vi "SetCategoryHierarchy.vi"(8 "error in (no error)":errorcluster, 9 "Category hierarchy[]":string[](array[string]), 11 "CLabVIEWItem in":refnum<class "CLabVIEWItem.lvclass">) -> (0 "error out":errorcluster, 3 "CLabVIEWItem out":refnum<class "CLabVIEWItem.lvclass">)   [LabVIEW 2020, in "LabVIEWItem.lvlib" / "CLabVIEWItem.lvclass"]
uses:
  CLabVIEWItem.lvclass
  CLabVIEWItem.lvclass/CLabVIEWItem.ctl
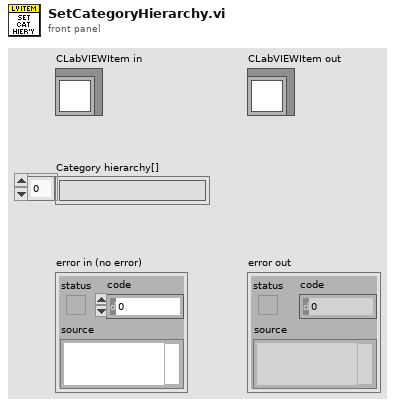
[diagram p1: front panel]
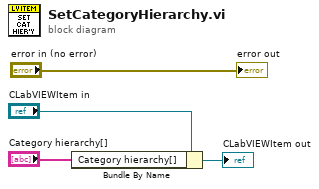
[diagram p0: block diagram]
diagram:
  n1 = Bundle By Name(cluster="CLabVIEWItem in", "Category hierarchy[]"="Category hierarchy[]") -> (→"CLabVIEWItem out":refnum<class "CLabVIEWItem.lvclass">)
  "error out" <- "error in (no error)"
